vi "Optionen Cluster Alle Anordnen.vi"(6 "Sprachliste":string[][](array[string]), 7 "Optionen":T1, 8 "error in (no error)":errorcluster caption="Fehler (Eingang, kein Fehler)", 11 "Cluster (Eingang)":refnum<vi>) -> (0 "error out":errorcluster caption="Fehler (Ausgang)", 3 "Numerisch":i32)   [LabVIEW 2020, in "System Einstellungen V2.lvlib"]
uses:
  System Einstellungen V2.lvlib
  Optionen.ctl
  Sprachverwaltung/Sprachverwaltung.lvlib
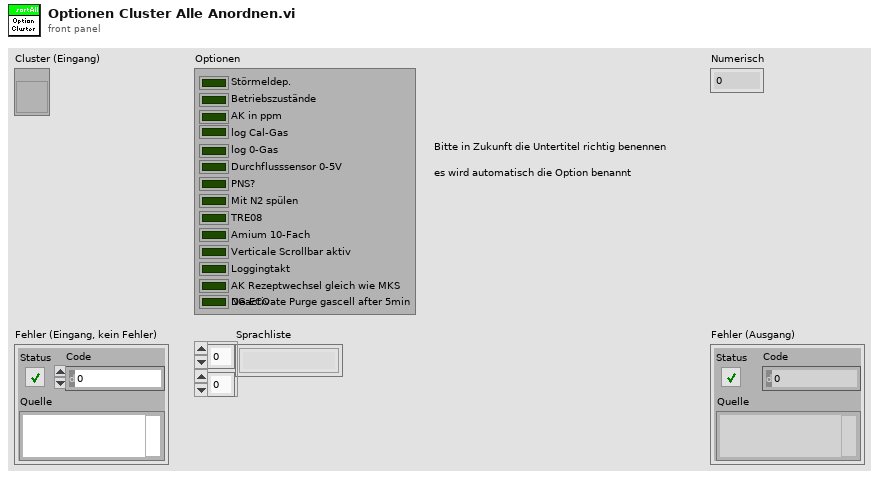
[diagram p1: front panel]
types:
  T1 = typedef "System Einstellungen V2.lvlib/Optionen.ctl" = cluster{"Störmeldep.":bool, "Betriebszustände":bool, "AK in ppm":bool, "log Cal-Gas":bool, "log 0-Gas":bool, "Durchflusssensor 0-5V":bool, "PNS?":bool, "Mit N2 spülen":bool, "TRE08":bool, "Amium 10-Fach":bool, "Verticale Scrollbar aktiv":bool, "Loggingtakt":bool, "AK Rezeptwechsel gleich wie MKS":bool, "NG ECO":bool}
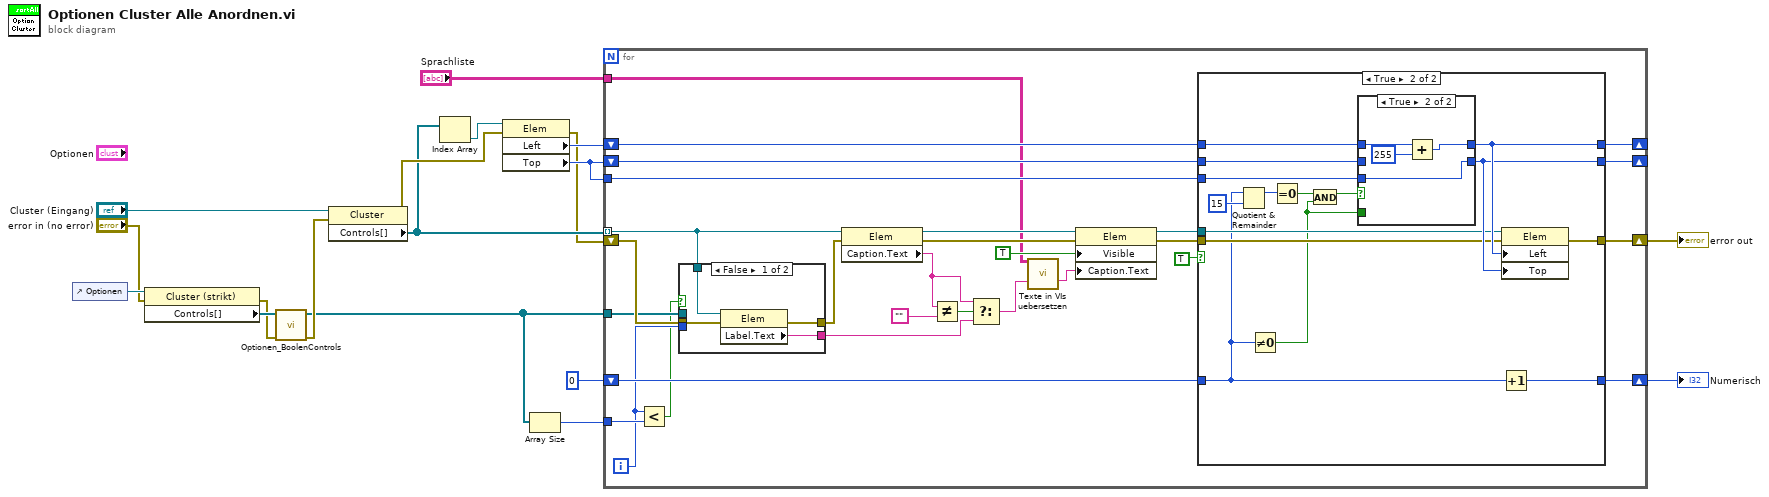
[diagram p0: block diagram]
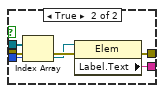
[diagram p2: hidden frame]
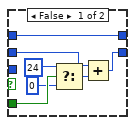
[diagram p4: hidden frame]
diagram:
  n1 = control-ref of="Optionen"() -> (w8:refnum<vi>)
  n2 = property class="Cluster (strikt)"(reference=w8, error in="error in (no error)") -> (error out=w4:errorcluster, "Controls[]"=w5:refnum<vi>[])  [unwired: 1 out]
  n3 = call "Optionen_BoolenControls.vi"("error in (no error)"=w4, "Controls[]"=w5) -> ("error out"=w3:errorcluster, "BooleanControls[] (Ausgang)"=w2:refnum<vi>[])  [unwired: 8 in]
  n4 = property class="Cluster"(reference="Cluster (Eingang)", error in=w3) -> (error out=w16:errorcluster, "Controls[]"=w15:refnum<vi>[])  [unwired: 1 out]
  n5 = Index Array(array=w15) -> (element=w17:refnum<vi>)  [unwired: 1 in]
  n6 = property class="Elem"(reference=w17, error in=w16) -> (error out=w11:errorcluster, "Left"=w14:i32, "Top"=w12:i32)  [unwired: 1 out]
  n7 = Array Size(array=w2) -> (size(s)=w6:i32)
  n8 = for {
    tunnel: w15 -> [w25] mode=indexing
    shift-right: [w46] -> w13
    shift-left: w11 -> [w29]
    shift-right: [w43] -> _
    shift-left: w14 -> [w45]
    shift-right: [w42] -> _
    shift-left: w12 -> [w44]
    tunnel: w12 -> [w41]
    shift-right: [w39] -> w9
    shift-left: 0 -> [w40]
    tunnel: w2 -> [w26]
    tunnel: w6 -> [w24]
    tunnel: "Sprachliste" -> [w19]
    i -> [w23]
    n9 = Less?(x=w23, y=w24) -> (x < y?=w22:bool)
    n10 = case shown="False" w22 {
      tunnel: w29 -> [w49 w56]
      tunnel: [w48 w55] -> w28
      tunnel: [w47 w54] -> w27
      tunnel: w26 -> [_ w52]
      tunnel: w23 -> [_ w51]
      tunnel: w25 -> [w50 _]
      frame False {
        n11 = property class="Elem"(reference=w50, error in=w49) -> (error out=w48:errorcluster, "Label.Text"=w47:string)  [unwired: 1 out]
      }
      frame True {
        n12 = Index Array(array=w52, index=w51) -> (element=w53:refnum<vi>)
        n13 = property class="Elem"(reference=w53, error in=w56) -> (error out=w55:errorcluster, "Label.Text"=w54:string)  [unwired: 1 out]
      }
    }
    n14 = property class="Elem"(reference=w25, error in=w28) -> (reference out=w33:refnum<vi>, error out=w34:errorcluster, "Caption.Text"=w30:string)
    n15 = Not Equal?(x=w30, y="") -> (x != y?=w31:bool)
    n16 = Select(t=w30, s=w31, f=w27) -> (s? t:f=w21:string)
    n17 = call "Texte in VIs uebersetzen.vi"("Sprachliste"=w19, "String zum Übersetzen"=w21) -> ("String zum Übersetzen"=w20:string)  [unwired: 9 in, 4 out]
    n18 = property class="Elem"(reference=w33, error in=w34, "Visible"=TRUE ("Sichtbar"), "Caption.Text"=w20) -> (reference out=w37:refnum<vi>, error out=w38:errorcluster)
    n19 = case shown="True" TRUE {
      tunnel: [w59 w75] -> w46
      tunnel: w45 -> [w58 w71]
      tunnel: w44 -> [w57 w70]
      tunnel: [w58 w69] -> w43
      tunnel: [w57 w68] -> w42
      tunnel: w41 -> [_ w67]
      tunnel: w40 -> [w60 w63]
      tunnel: [w60 w66] -> w39
      tunnel: w38 -> [w59 w65]
      tunnel: w37 -> [_ w64]
      frame False {
      }
      frame True {
        n20 = Quotient & Remainder(x=w63, y=15) -> (x-y*floor(x/y)=w73:i32)  [unwired: 1 out]
        n21 = Not Equal To 0?(x=w63) -> (x != 0?=w61:bool)
        n22 = Equal To 0?(x=w73) -> (x = 0?=w72:bool)
        n23 = And(x=w72, y=w61) -> (x .and. y?=w62:bool)
        n24 = case shown="True" w62 {
          tunnel: w71 -> [w82 w85]
          tunnel: w70 -> [w81 _]
          tunnel: [w82 w83] -> w69
          tunnel: [w80 w86] -> w68
          tunnel: w67 -> [_ w86]
          tunnel: w61 -> [w78 _]
          frame False {
            n25 = Select(t=24 ("y"), s=w78, f=0) -> (s? t:f=w79:i32)
            n26 = Add(x=w81, y=w79) -> (x+y=w80:i32)
          }
          frame True {
            n27 = Add(x=w85, y=255) -> (x+y=w83:i32)
          }
        }
        n28 = Increment(x=w63) -> (x+1=w66:i32)
        n29 = property class="Elem"(reference=w64, error in=w65, "Left"=w69, "Top"=w68) -> (error out=w75:errorcluster)  [unwired: 1 out]
      }
    }
  }
  "error out" <- w13
  "Numerisch" <- w9
